vi "RT Audio Filter Matlab Node.vi"() -> ()   [LabVIEW 2022 SP3]
uses:
  <vilib>/Analysis/3filter.llb/Filter Passband Type.ctl
  <vilib>/FPGAPlugInAG/myRIO-1900/niLvFpga_Open_myRIO-1900.vi
  <vilib>/rvi/interface/common/dynamic/niFpgaDynamicAddResources.vi
  <vilib>/Utility/error.llb/Error Cluster From Error Code.vi
  <vilib>/rvi/errors/niLvFpgaAdjustHostInterfaceError.vi
  <vilib>/Analysis/3filter.llb/Butterworth Filter (DBL).vi
  <vilib>/imath/engines/lvmath2/RunTimeEngine/BuiltInFunctions/iir_butterord/NIMS_iir_butterord.vi
  <vilib>/imath/engines/lvmath2/RunTimeEngine/ErrorHandling/NIMS_Create Error From Enums.vi
  <vilib>/imath/engines/lvmath2/RunTimeEngine/BuiltInFunctions/iir_butter/NIMS_[2o]_iir_butter(I32,V).vi
  <vilib>/imath/engines/lvmath2/RunTimeEngine/ErrorHandling/NIMS_Error From Error Code.vi
  <vilib>/imath/engines/lvmath2/RunTimeEngine/BuiltInFunctions/filter/NIMS_filter(GV,GV,GV,GV,Str).vi
  <instcachedir>/0/NIMS_filter(GV,GV,GV,GV,Str)_7C5B88D942D8486E8E164CAC1589CA58.lvgen/NIMS_filter(GV,GV,GV,GV,Str)_7C5B88D942D8486E8E164CAC1589CA58_000.vi
  <vilib>/imathl/engines/lvmath/Functions/Error Handling/Create Error.vi
  <vilib>/imath/engines/lvmath2/RunTimeEngine/BuiltInFunctions/iir_butter/NIMS_[2o]_iir_butter(I32,V,Str).vi
  <vilib>/imath/engines/lvmath2/RunTimeEngine/NodeEndStatement/NIMS_NodeEndStatement_Output.vi
  <instcachedir>/0/NIMS_NodeEndStatement_Output_53EC0D466D134D7ABD903AC30B43404B.lvgen/NIMS_NodeEndStatement_Output_53EC0D466D134D7ABD903AC30B43404B_005.vi
  <vilib>/imath/engines/lvmath2/RunTimeEngine/ErrorHandling/NIMS_Finalize Error.vi
  <vilib>/FPGAPlugInAG/Dynamic/niLvFpga_Close_Dynamic.vi
  <vilib>/rvi/interface/nirviOpenFPGA/nirviOpenFPGA.xnode
  FPGA Bitfiles/FPGA Audio Streaming (with LEDs).lvbitx
  FPGA Audio Streaming.vi
  <vilib>/rvi/interface/nirviReadWriteControl/nirviReadWriteControl.xnode
  <vilib>/rvi/interface/nirviCloseFPGA/nirviCloseFPGA.xnode
  <vilib>/Analysis/NI_AALBase.lvlib
  <vilib>/rvi/interface/Simulation/niFpgaSimulationCallBeginRW.vi
  NiFpgaLv.dll
panel:
  in  "Base":dbl(slide) scale=0.0..1.0
  in  "Mode Select":bool
  in  "Midtone":dbl(slide)=1.0 scale=0.0..1.0
  in  "Treble":dbl(slide)=1.0 scale=0.0..1.0
  out "Model of Computation":string
  in  "Sample Rate (Hz)":dbl=44101.0
  out "Audio Spectrum":dynamicdata(graph)
  in  "Read Rate (Hz)":dbl=5.0
  in  "stop":bool
  # "Audio Equilizer Control"
  # "Application Control"
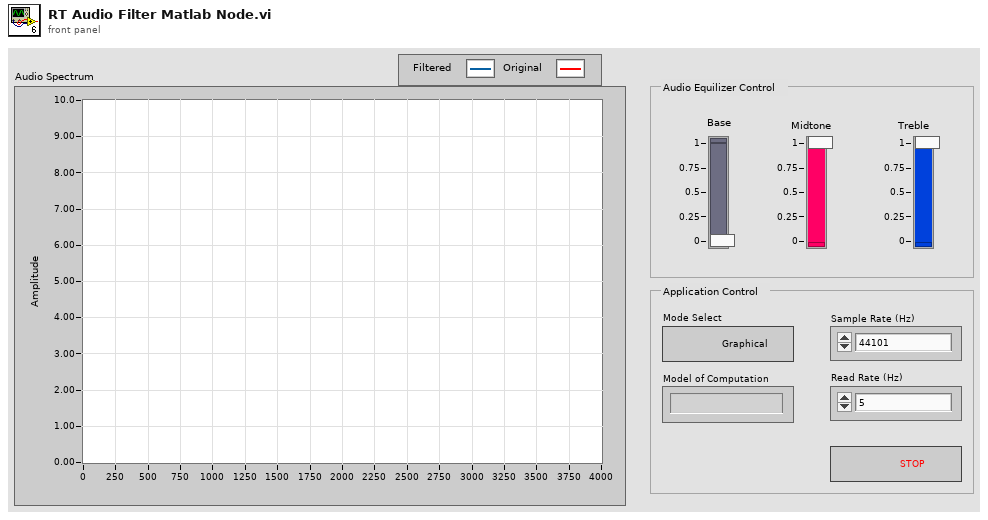
[diagram p1: front panel]
types:
  T1 = typedef "NI_AALBase.lvlib/Filter Passband Type.ctl" = enum32{"Lowpass", "Highpass", "Bandpass", "Bandstop"}
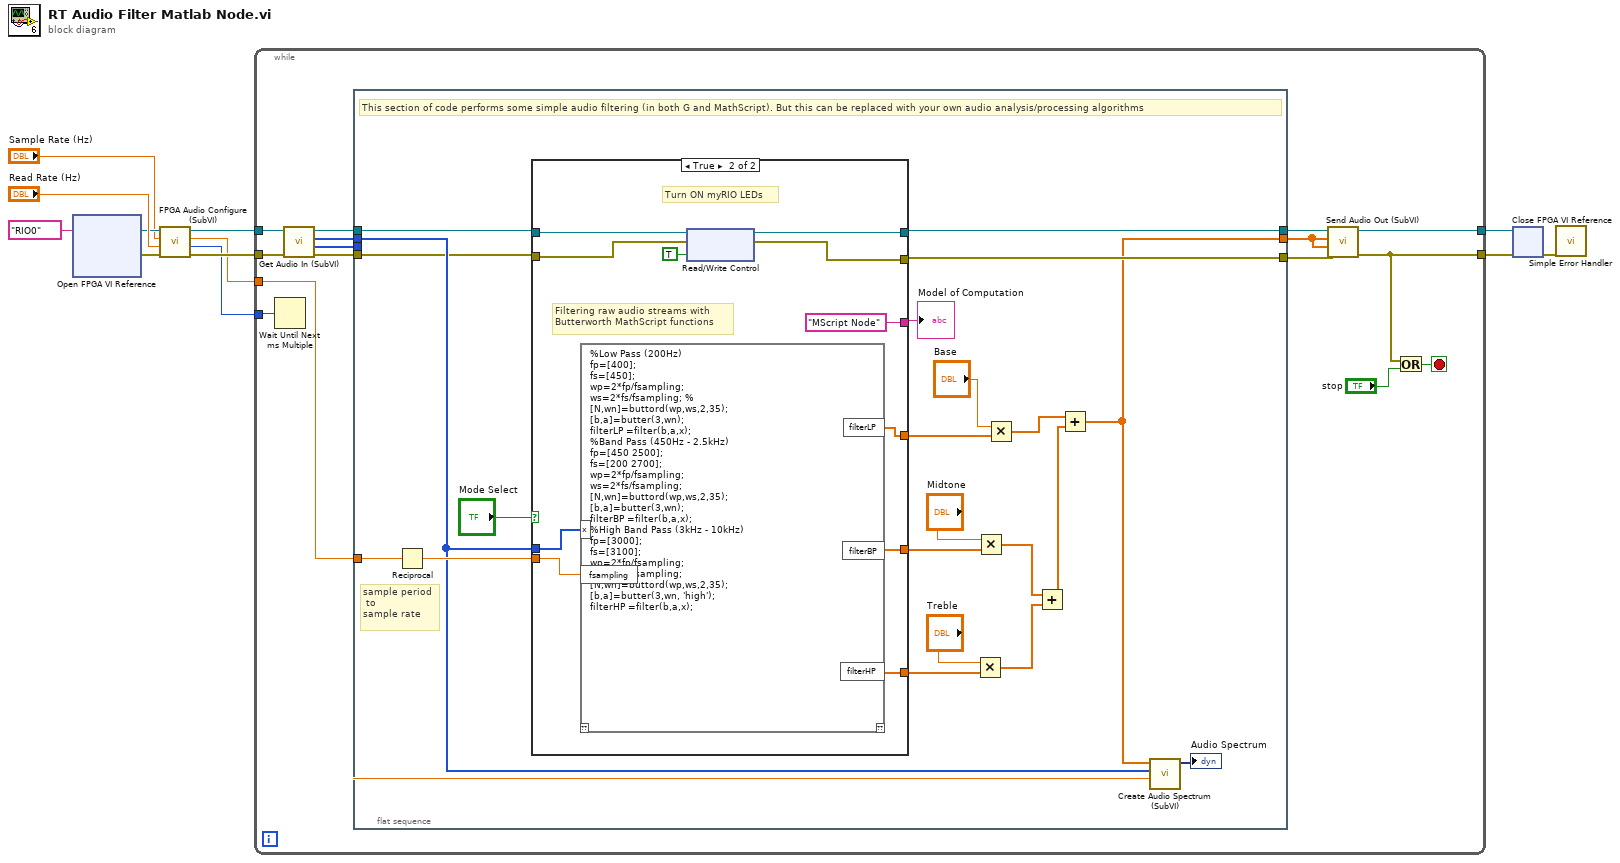
[diagram p0: block diagram]
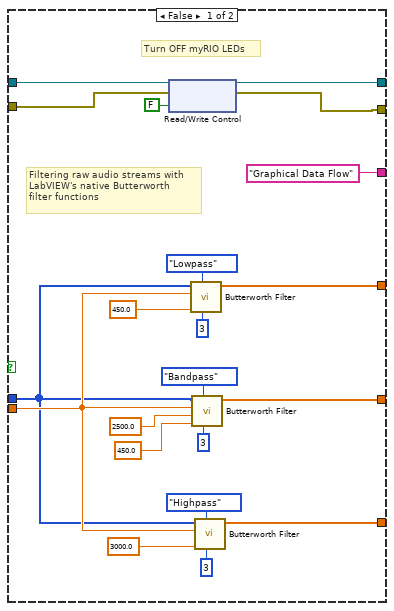
[diagram p2: hidden frame]
diagram:
  n1 = xnode "Open FPGA VI Reference"("resource name"=tag "RIO0") -> ("FPGA VI Reference Out"=w5:refnum<k20>, "error out"=w12:errorcluster)  [unwired: 1 in]
  n2 = call "FPGA Audio Configure (SubVI).vi"("error in (no error)"=w12, "Read Rate (Hz)"="Read Rate (Hz)", "Audio Sample Rate (Hz)"="Sample Rate (Hz)", "Refnum in"=w5) -> ("error out"=w7:errorcluster, "Required loop period (ms)"=w2:u32, "Audio dt (ms)"=w3:dbl, "Refnum out"=w11:refnum<k20>)  [unwired: 4 in]
  n3 = while {
    tunnel: w11 -> [w24]
    tunnel: [w22] -> w10
    tunnel: [w18] -> w9
    tunnel: w2 -> [w23]
    tunnel: w7 -> [w25]
    tunnel: w3 -> [w21]
    stop <- w26 stop-if-true
    n4 = Wait Until Next ms Multiple(millisecond multiple=w23) -> ()  [unwired: 1 out]
    n5 = call "Get Audio In (SubVI).vi"("error in (no error)"=w25, "Refnum in"=w24) -> ("error out"=w16:errorcluster, "Right Audio In"=w13:i16[], "Left Audio In"=w19:i16[], "Refnum out"=w17:refnum<k20>)  [unwired: 6 in]
    n6 = flat-sequence {
      tunnel: w21 -> [w41]
      tunnel: [w30] -> w20
      tunnel: w19 -> [w37]
      tunnel: w17 -> [w36]
      tunnel: w16 -> [w35]
      tunnel: [w34] -> w15
      tunnel: [w33] -> w14
      tunnel: w13 -> [_]
      frame #0 {
        # "sample period\n to\nsample rate"
        # "This section of code performs some simple audio filtering (in both G and MathScript). But this can be replaced with your own audio analysis/processing algorithms"
        n7 = Reciprocal(x=w41) -> (1/x=w48:dbl)
        n8 = case shown="True" "Mode Select" {
          tunnel: [w67 w79] -> w43
          tunnel: [w66 w80] -> w42
          tunnel: ["Graphical Data Flow" ("Mode") "MScript Node" ("Mode")] -> w40
          tunnel: w48 -> [w59 w77]
          tunnel: w37 -> [w55 w76]
          tunnel: w36 -> [w54 w75]
          tunnel: w35 -> [w53 w74]
          tunnel: [w51 w72] -> w34
          tunnel: [w52 w71] -> w33
          tunnel: [w49 w70] -> w32
          frame False {
            # "Turn OFF myRIO LEDs"
            # "Filtering raw audio streams with \nLabVIEW's native Butterworth \nfilter functions"
            n9 = xnode "Read/Write Control"("FPGA VI Reference In"=w54, "error in"=w53, "LEDs On?"=FALSE) -> ("FPGA VI Reference Out"=w51:refnum<k20>, "error out"=w52:errorcluster)
            n10 = call-poly <vilib>:"Butterworth Filter.vi"("order"=3, "filter type"=Filter_Passband_Type."Lowpass", "low cutoff freq: fl"=450.0, "sampling freq: fs"=w59, "X"=w55) -> ("Filtered X"=w49:dbl[])  [unwired: 3 in, 1 out]
            n11 = call-poly <vilib>:"Butterworth Filter.vi"("order"=3, "filter type"=Filter_Passband_Type."Bandpass", "low cutoff freq: fl"=450.0, "high cutoff freq: fh"=2500.0, "sampling freq: fs"=w59, "X"=w55) -> ("Filtered X"=w67:dbl[])  [unwired: 2 in, 1 out]
            n12 = call-poly <vilib>:"Butterworth Filter.vi"("order"=3, "filter type"=Filter_Passband_Type."Highpass", "low cutoff freq: fl"=3000.0 ("high cutoff freq: fh"), "sampling freq: fs"=w59, "X"=w55) -> ("Filtered X"=w66:dbl[])  [unwired: 3 in, 1 out]
          }
          frame True {
            # "Turn ON myRIO LEDs"
            # "Filtering raw audio streams with \nButterworth MathScript functions"
            n13 = mathscript code="%Low Pass (200Hz)\nfp=[400]; \nfs=[450]; \nwp=2*fp/fsampling; \nws=2*fs/fsampling; %\n[N,wn]=buttord(wp,ws,2,35);\n[b,a]=butter(3,wn);\nfilterLP =filter(b,a,x);\n%Band Pass (450Hz - 2.5kHz)\nfp=[450 2500]; \nfs=[200 2700]; \nwp=2*fp/fsampling; \nws=2*fs/fsampling; \n[N,wn]=buttord(wp,ws,2,35);\n[b,a]=butter(3,wn);\nfilterBP =filter(b,a,x);\n%High Band Pass (3kHz - 10kHz)\nfp=[3000]; \nfs=[3100]; \nwp=2*fp/fsampling; \nws=2*fs/fsampling; \n[N,wn]=buttord(wp,ws,2,35);\n[b,a]=butter(3,wn, 'high');\nfilterHP =filter(b,a,x);"("x"=w76, "fsampling"=w77) -> ("filterBP"=w79:dbl[], "filterHP"=w80:dbl[], "filterLP"=w70:dbl[])  [unwired: 1 in, 1 out]
            n14 = xnode "Read/Write Control"("FPGA VI Reference In"=w75, "error in"=w74, "LEDs On?"=TRUE) -> ("FPGA VI Reference Out"=w72:refnum<k20>, "error out"=w71:errorcluster)
          }
        }
        "Model of Computation" <- w40
        n15 = Multiply(x="Treble", y=w42) -> (x*y=w44:dbl[])
        n16 = Multiply(x="Midtone", y=w43) -> (x*y=w45:dbl[])
        n17 = Multiply(x="Base", y=w32) -> (x*y=w29:dbl[])
        n18 = Add(x=w45, y=w44) -> (x+y=w31:dbl[])
        n19 = Add(x=w29, y=w31) -> (x+y=w30:dbl[])
        n20 = call "Create Audio Spectrum (SubVI).vi"("Sample Period (ms)"=w41, "Raw Audio"=w37, "Filtered Audio"=w30) -> ("FFT Out"=→"Audio Spectrum":dynamicdata)  [unwired: 8 in]
      }
    }
    n21 = call "Send Audio Out (SubVI).vi"("error in (no error)"=w14, "Right Audio Out"=w20, "Left Audio Out"=w20, "Refnum in"=w15) -> ("error out"=w18:errorcluster, "Refnum out"=w22:refnum<k20>)  [unwired: 6 in]
    n22 = Or(x=w18, y="stop") -> (x .or. y?=w26:bool)
  }
  n23 = xnode "Close FPGA VI Reference"("FPGA VI Reference In"=w10, "error in"=w9) -> ("error out"=w1:errorcluster)
  n24 = call <vilib>:"Simple Error Handler.vi"("error in (no error)"=w1) -> ()  [unwired: 4 in, 5 out]
